vi "create default alias.vi"(8 "error in":errorcluster, 11 "configuration in":refnum<class "TDMS datalogger configuration.lvclass">) -> (0 "error out":errorcluster, 2 "default alias":string, 3 "configuration out":refnum<class "TDMS datalogger configuration.lvclass">)   [LabVIEW 2015, in "TDMS datalogger configuration.lvclass"]
uses:
  TDMS datalogger configuration.lvclass
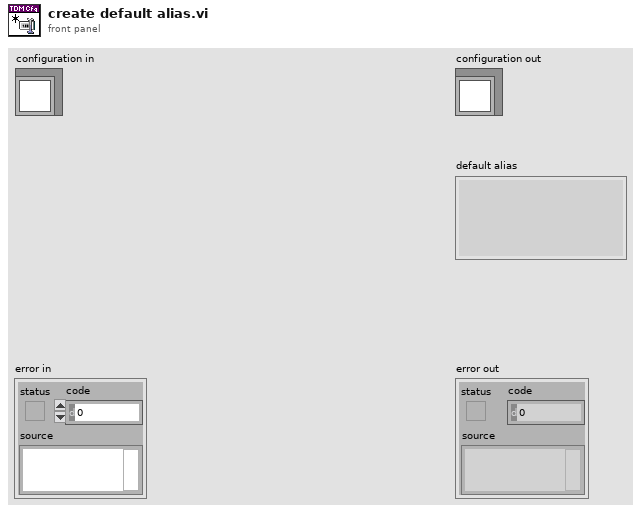
[diagram p1: front panel]
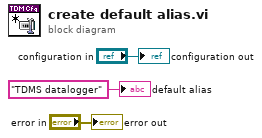
[diagram p0: block diagram]
diagram:
  "error out" <- "error in"
  "configuration out" <- "configuration in"
  "default alias" <- "TDMS datalogger" ("default alias")
